vi "Init.vi"(7 "I2C #":T2=-1, 8 "error in (no error)":errorcluster, 9 "Address":T1 format="%02x", 10 "Session In":refnum<class "Session.lvclass">) -> (0 "error out":errorcluster, 3 "4ChannelSPDTRelay Out":refnum<class "4ChannelSPDTRelay.lvclass">)   [LabVIEW 2020, in "CTI-Peripheral.lvlib" / "4ChannelSPDTRelay.lvclass"]
uses:
  4ChannelSPDTRelay.lvclass
  CTI/Session/Session.lvclass
  CTI/I2C Number.ctl
  CTI/I2C Address.ctl
  CTI/I2C Connection/I2C Connection.lvclass/I2C Connection.ctl
  4ChannelSPDTRelay.lvclass/4ChannelSPDTRelay.ctl
  CTI/I2C Connection/I2C Connection.lvclass
  CTI/CTI.lvlib
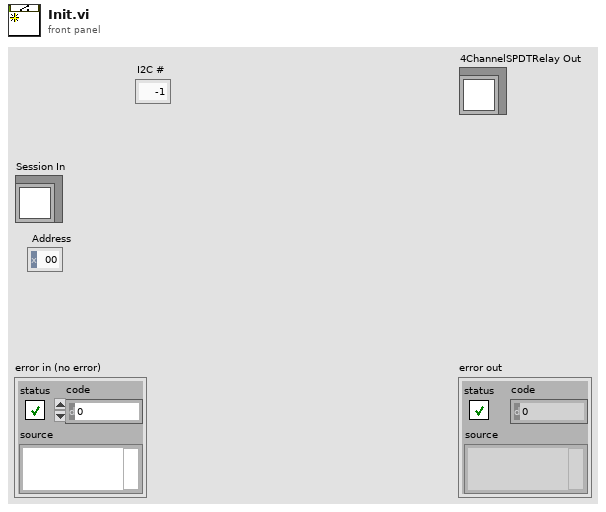
[diagram p1: front panel]
types:
  T1 = typedef "CTI.lvlib/I2C Address.ctl" = u8
  T2 = typedef "CTI.lvlib/I2C Number.ctl" = i8
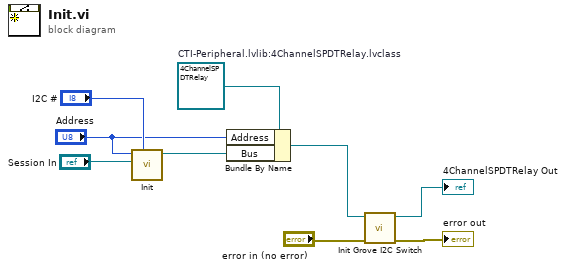
[diagram p0: block diagram]
diagram:
  w1 = refnum<class "4ChannelSPDTRelay.lvclass"> refnum  # CTI-Peripheral.lvlib:4ChannelSPDTRelay.lvclass
  n1 = call "Init.vi"("I2C #"="I2C #", "Session"="Session In", "Address"="Address") -> ("I2C Connection"=w9:refnum<class "I2C Connection.lvclass">)  [unwired: 7 in, 1 out]
  n2 = Bundle By Name(cluster=w1, "Address"="Address", "Bus"=w9) -> (w4:refnum<class "4ChannelSPDTRelay.lvclass">)
  n3 = call "Init Grove I2C Switch.vi"("error in (no error)"="error in (no error)", "I2C RGB SGM31323 in"=w4) -> ("error out"=→"error out":errorcluster, "I2C RGB SGM31323 out"=→"4ChannelSPDTRelay Out":refnum<class "4ChannelSPDTRelay.lvclass">)  [unwired: 8 in]
